vi "Get 2D Array Double Complex.vi"(5 "use temporary file? (F)":bool, 7 "data type of variable":cdb[][](array[numeric]), 8 "error in":errorcluster, 10 "variable name":string, 11 "GOLPI ref. in":T1={"pipe handle"={"lv_proc.dll file path"=path "", "process instance handle"=[], "debug mode"=FALSE, "debug data"=[]}, "fast read timeout [ms]"=500, "fast read settle time [ms]"=10, "fast read to multiple [ms]"=1, "max elements per input line"=100, "slow read timeout [ms]"=5000, "stdin double format specifier"="%_16e", "max elements per stdout output column"=100, "console mode bitstream"=FALSE, "bitstream first read timeout [ms]"=1000, "bitstream read timeout [ms]"=50, "struct transfer possible"=FALSE}) -> (0 "error out":errorcluster, 2 "value":cdb[][](array[numeric]) format="%.2f", 3 "GOLPI ref. out":T1={"pipe handle"={"lv_proc.dll file path"=path "", "process instance handle"=[], "debug mode"=FALSE, "debug data"=[]}, "fast read timeout [ms]"=500, "fast read settle time [ms]"=10, "fast read to multiple [ms]"=1, "max elements per input line"=100, "slow read timeout [ms]"=5000, "stdin double format specifier"="%_16e", "max elements per stdout output column"=100, "console mode bitstream"=FALSE, "bitstream first read timeout [ms]"=1000, "bitstream read timeout [ms]"=50, "struct transfer possible"=FALSE})   [LabVIEW 2013, in "GOLPI library.lvlib"]
doc: "Part of polymorph Get Variable.vi"
uses:
  GOLPI library.lvlib
  Public/GOLPI reference Type Def.ctl
  LV Process source distribution/Pipe Handle.ctl
  Type Definitions/Bitstream Data Type.ctl
  Type Definitions/Custom Error Codes Enum Type Def.vi
  LV Process source distribution/LV Process library.lvlib
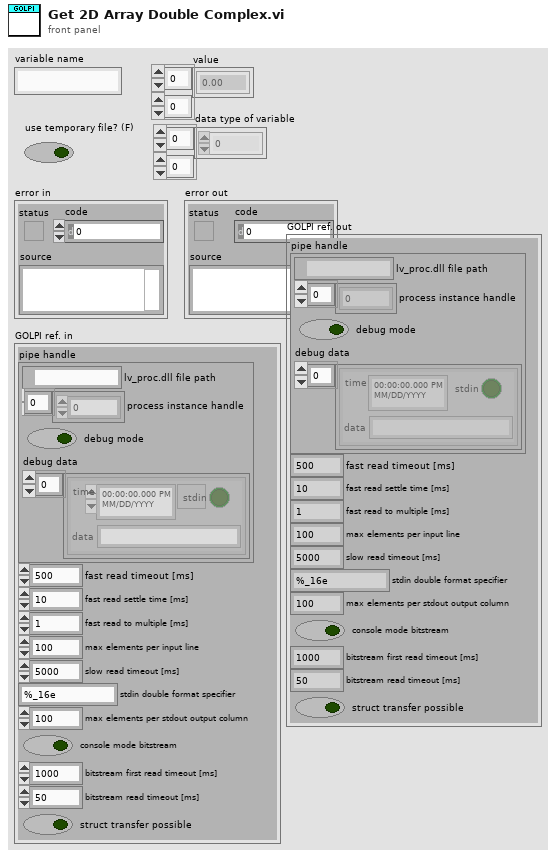
[diagram p1: front panel]
types:
  T1 = typedef "GOLPI library.lvlib/GOLPI reference Type Def.ctl" = cluster{"pipe handle":T2, "fast read timeout [ms]":u32, "fast read settle time [ms]":u32, "fast read to multiple [ms]":u32, "max elements per input line":u32, "slow read timeout [ms]":u32, "stdin double format specifier":string, "max elements per stdout output column":u32, "console mode bitstream":bool, "bitstream first read timeout [ms]":u32, "bitstream read timeout [ms]":u32, "struct transfer possible":bool}
  T2 = typedef "LV Process library.lvlib/Pipe Handle.ctl" = cluster{"lv_proc.dll file path":path, "process instance handle":u32[], "debug mode":bool, "debug data":cluster{"time":timestamp, "stdin":bool, "data":string}[]}
  T3 = typedef "GOLPI library.lvlib/Bitstream Data Type.ctl" = enum16{"dummy", "int", "uint", "float", "complex", "str", "real numeric"}
  T4 = typedef "GOLPI library.lvlib/Custom Error Codes Enum Type Def.vi" = enum16{"no error", "00 working directory PAR1 missing", "01 octave binary PAR1 missing", "02 octave report error PAR1", "03 empty output last cmd PAR1", "04 missing temporary file PAR1", "05 pwd PAR 1 not exist", "10 var PAR1 not string, vect", "11 var PAR1 not num, scal, ~compl", "12 var PAR1 not num, scal, compl", "13 var PAR1 not num, vect, ~compl", "14 var PAR1 not num, vect, compl", "15 var PAR1 not num, mat, ~compl", "16 var PAR1 not num, mat, ~compl", "30 read timeout", "60 bitstream transport failed", "61 bitstream decode error PAR1", "62 bitstream cannot be set", "70 struct transfer not possible", "80 struct: cluster elem. PAR1 not implem.", "81 struct: structure field PAR1 not implem.", "82 struct: size mismatch of PAR1", "83 struct: type mismatch of PAR1", "98 internal error", "99 not finished"}
  T5 = typedef "GOLPI library.lvlib/Bitstream Data.ctl" = cluster{"double":dbl[][], "cplx double":cdb[][], "int64":i64[][], "uint64":u64[][], "str":string[], "data type":T3}
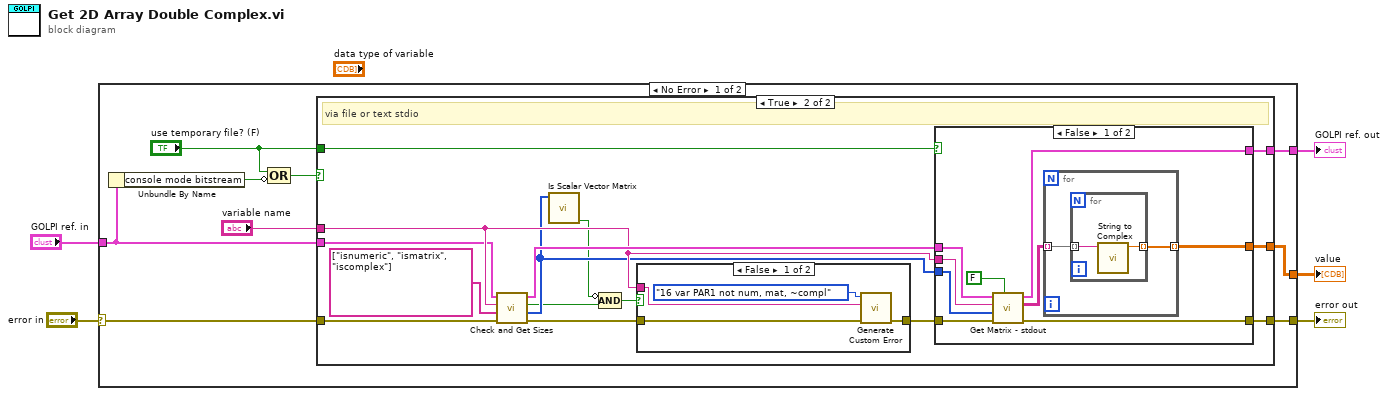
[diagram p0: block diagram]
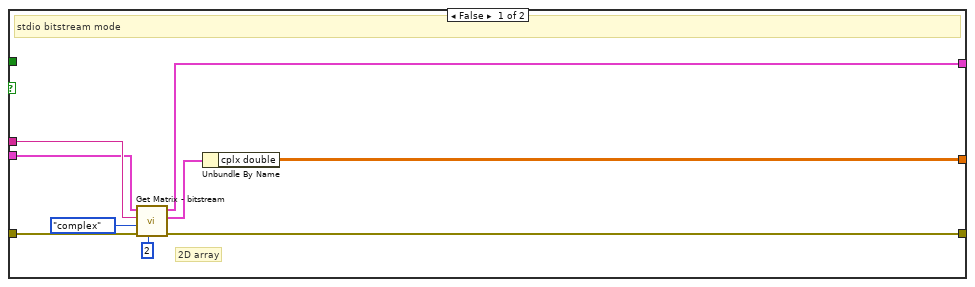
[diagram p2: hidden frame]
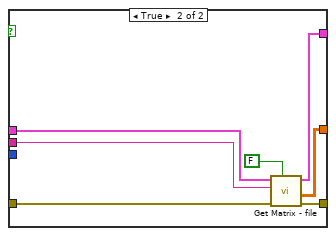
[diagram p3: hidden frame]
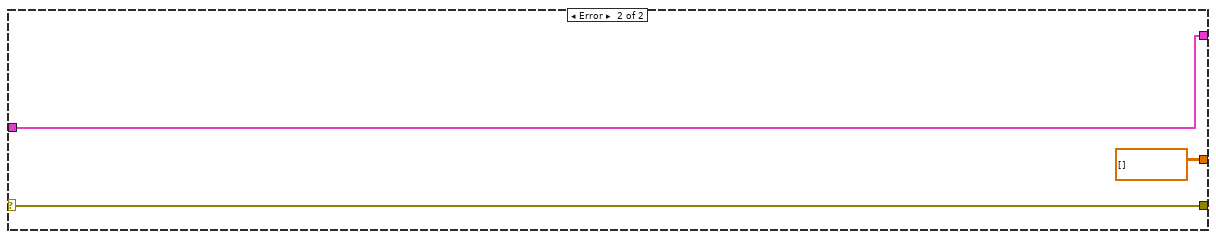
[diagram p5: hidden frame]
diagram:
  n1 = case shown="No Error" "error in" {
    selector: "error in" -> [w14 w66]
    tunnel: [w13 w66] -> w5
    tunnel: [w11 cdb[][] [] ("value")] -> w3
    tunnel: "GOLPI ref. in" -> [w9 w64]
    tunnel: [w10 w64] -> w1
    frame No Error {
      n2 = Unbundle By Name(w9) -> ("console mode bitstream"=w8:bool)
      n3 = Compound Arithmetic op=OR("use temporary file? (F)", invert w8) -> (w6:bool)
      n4 = case shown="True" w6 {
        tunnel: w14 -> [w23 w38]
        tunnel: [w17 w33] -> w13
        tunnel: "variable name" -> [w22 w32]
        tunnel: "use temporary file? (F)" -> [_ w31]
        tunnel: [w15 w30] -> w11
        tunnel: w9 -> [w19 w29]
        tunnel: [w18 w28] -> w10
        frame False {
          # "2D array"
          # "stdio bitstream mode"
          n5 = call "Get Matrix - bitstream.vi"("max dimensions (0: scalar)"=2, "error in (no error)"=w23, "data type"=Bitstream_Data_Type."complex", "variable name"=w22, "GOLPI ref. in"=w19) -> ("error out"=w17:errorcluster, "data"=w16:T5, "GOLPI ref. out"=w18:T1)  [unwired: 4 in]
          n6 = Unbundle By Name(w16) -> ("cplx double"=w15:cdb[][])
        }
        frame True {
          # "via file or text stdio"
          n7 = call "Check and Get Sizes.vi"("error in (no error)"=w38, "test commands"=string[] ["isnumeric", "ismatrix", "iscomplex"], "variable name"=w32, "GOLPI ref. in"=w29) -> ("error out"=w37:errorcluster, "octave sizes"=w27:i32[], "all tests OK?"=w26:bool, "GOLPI ref. out"=w35:T1)  [unwired: 4 in]
          n8 = call "Is Scalar Vector Matrix.vi"("octave sizes"=w27) -> ("is >2d matrix?"=w24:bool)  [unwired: 5 in, 5 out]
          n9 = Compound Arithmetic op=AND(invert w24, w26) -> (w25:bool)
          n10 = case shown="False" w25 {
            tunnel: w37 -> [w61 w63]
            tunnel: [w60 w63] -> w34
            tunnel: w32 -> [w59 _]
            frame False {
              n11 = call "Generate Custom Error.vi"("error in"=w61, "PAR1"=w59, "GOLPI error"=Custom_Error_Codes_Enum_Type_Def.vi."16 var PAR1 not num, mat, ~compl" ("Enum")) -> ("error out"=w60:errorcluster)  [unwired: 8 in]
            }
            frame True {
            }
          }
          n12 = case shown="False" w31 {
            tunnel: w35 -> [w45 w54]
            tunnel: [w44 w55] -> w28
            tunnel: w34 -> [w42 w57]
            tunnel: [w43 w56] -> w33
            tunnel: w32 -> [w40 w53]
            tunnel: [w41 w52] -> w30
            tunnel: w27 -> [w39 _]
            frame False {
              n13 = call "Get Matrix - stdout.vi"("is string?"=FALSE ("is string"), "error in (no error)"=w42, "octave sizes"=w39, "variable name"=w40, "GOLPI ref. in"=w45) -> ("error out"=w43:errorcluster, "array"=w46:string[][], "GOLPI ref. out"=w44:T1)  [unwired: 4 in]
              n14 = for {
                tunnel: w46 -> [w49] mode=indexing
                tunnel: [w48] -> w41 mode=indexing
                n15 = for {
                  tunnel: w49 -> [w51] mode=indexing
                  tunnel: [w50] -> w48 mode=indexing
                  n16 = call "String to Complex.vi"("string"=w51) -> ("complex number"=w50:cdb)  [unwired: 10 in]
                }
              }
            }
            frame True {
              n17 = call "Get Matrix - file.vi"("is string?"=FALSE ("is string"), "error in (no error)"=w57, "variable name"=w53, "GOLPI ref. in"=w54) -> ("error out"=w56:errorcluster, "cmplx double array"=w52:cdb[][], "GOLPI ref. out"=w55:T1)  [unwired: 3 in, 2 out]
            }
          }
        }
      }
    }
    frame Error {
    }
  }
  "value" <- w3
  "error out" <- w5
  "GOLPI ref. out" <- w1
